vi "Display Item Info.vi"(8 "error in (no error)":errorcluster, 9 "Config":T1, 10 "Control References":T5, 11 "Item in":refnum<class "Item.lvclass">) -> (0 "error out":errorcluster, 3 "Item out":refnum<class "Item.lvclass">)   [LabVIEW 2020, in "VI Properties Editor.lvlib" / "Item.lvclass"]
doc: "Displays the data of <B>Item in</B> to the controls identified by <B>Control References</B>, taking into account <B>Config</B>."
uses:
  Item.lvclass
  CTLs/Main References.ctl
  CTLs/Config.ctl
  CTLs/Filter Info.ctl
  CTLs/Filter Column.ctl
  CTLs/Filter Type.ctl
  VI Properties Editor.lvlib
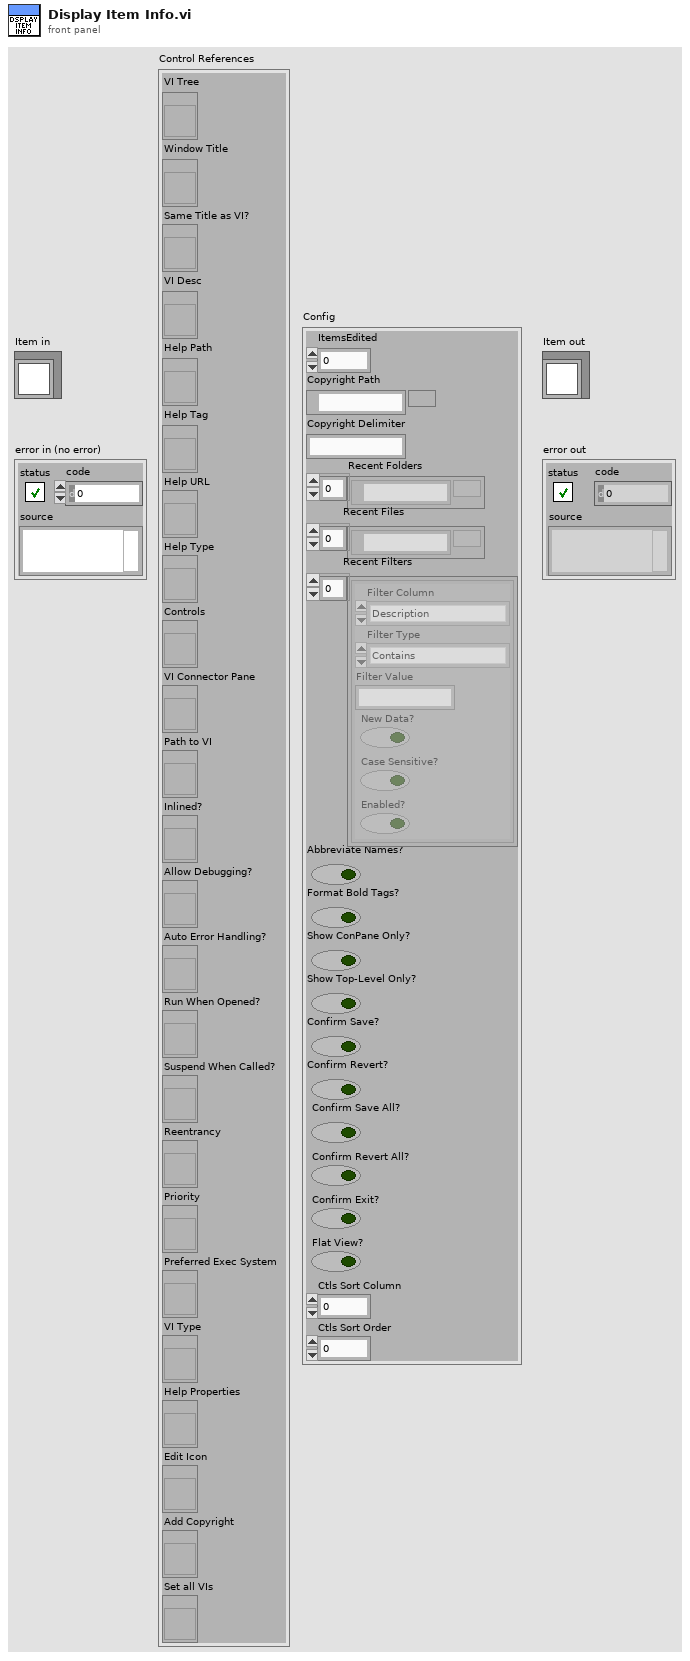
[diagram p1: front panel]
types:
  T1 = typedef "VI Properties Editor.lvlib/Config.ctl" = cluster{"ItemsEdited":u32, "Copyright Path":path, "Copyright Delimiter":string, "Recent Folders":path[], "Recent Files":path[], "Recent Filters":T2[], "Abbreviate Names?":bool, "Format Bold Tags?":bool, "Show ConPane Only?":bool, "Show Top-Level Only?":bool, "Confirm Save?":bool, "Confirm Revert?":bool, "Confirm Save All?":bool, "Confirm Revert All?":bool, "Confirm Exit?":bool, "Flat View?":bool, "Ctls Sort Column":i32, "Ctls Sort Order":i32}
  T2 = typedef "VI Properties Editor.lvlib/Filter Info.ctl" = cluster{"Filter Column":T3, "Filter Type":T4, "Filter Value":string, "New Data?":bool, "Case Sensitive?":bool, "Enabled?":bool}
  T3 = typedef "VI Properties Editor.lvlib/Filter Column.ctl" = enum16{"Name", "Path", "Type", "Window Title", "Description", "Help Path", "Help Tag", "Custom Title?", "Reentrancy", "Inlined?", "Help URL", "Help Type", "Allow Debugging?", "Auto Error Handling?", "Run When Opened?", "Suspend When Called?", "Priority", "Preferred Exec Sytem", "Control Label", "Control Caption", "Control Description", "Control Tip Strip"}
  T4 = typedef "VI Properties Editor.lvlib/Filter Type.ctl" = enum16{"Contains", "Equals", "Starts with", "Ends with", "Is empty", "Does not contain", "Does not equal", "Is not empty"}
  T5 = typedef "VI Properties Editor.lvlib/Main References.ctl" = cluster{"VI Tree":refnum<vi>, "Window Title":refnum<vi>, "Same Title as VI?":refnum<vi>, "VI Desc":refnum<vi>, "Help Path":refnum<vi>, "Help Tag":refnum<vi>, "Help URL":refnum<vi>, "Help Type":refnum<vi>, "Controls":refnum<vi>, "VI Connector Pane":refnum<vi>, "Path to VI":refnum<vi>, "Inlined?":refnum<vi>, "Allow Debugging?":refnum<vi>, "Auto Error Handling?":refnum<vi>, "Run When Opened?":refnum<vi>, "Suspend When Called?":refnum<vi>, "Reentrancy":refnum<vi>, "Priority":refnum<vi>, "Preferred Exec System":refnum<vi>, "VI Type":refnum<vi>, "Help Properties":refnum<vi>, "Edit Icon":refnum<vi>, "Add Copyright":refnum<vi>, "Set all VIs":refnum<vi>}
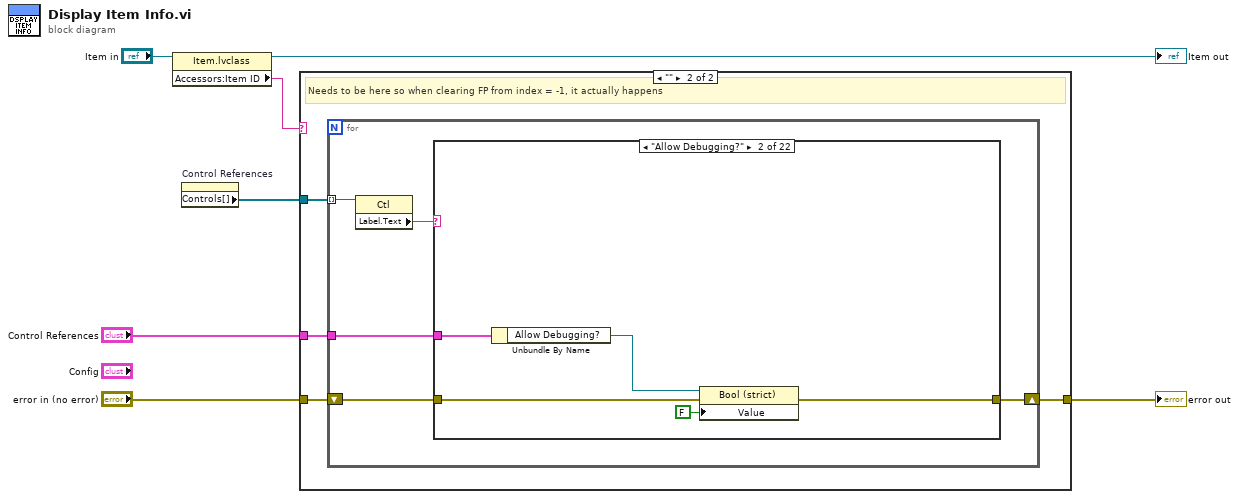
[diagram p0: block diagram]
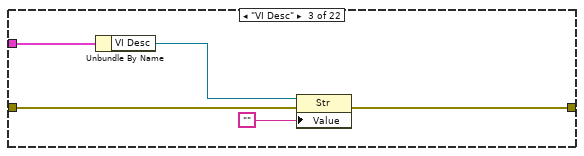
[diagram p4: hidden frame]
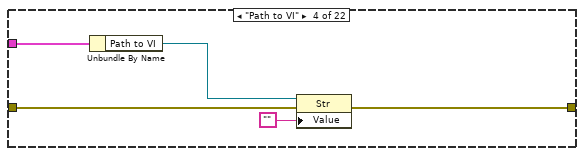
[diagram p5: hidden frame]
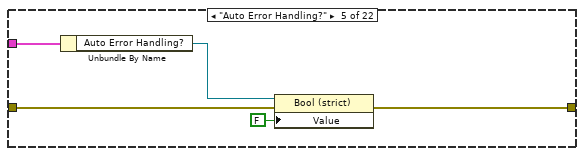
[diagram p6: hidden frame]
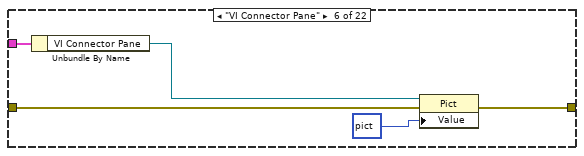
[diagram p7: hidden frame]
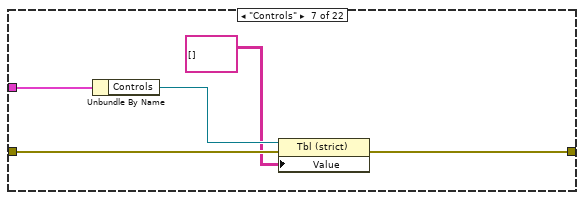
[diagram p8: hidden frame]
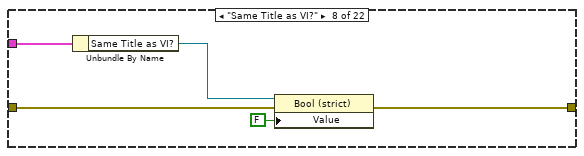
[diagram p9: hidden frame]
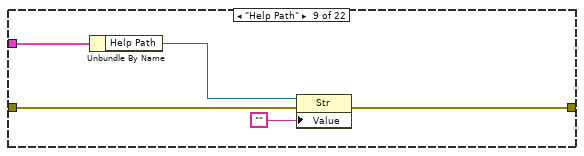
[diagram p10: hidden frame]
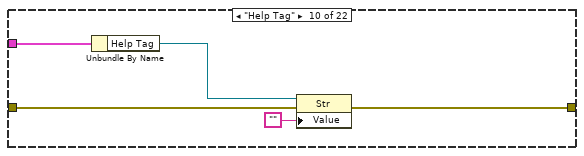
[diagram p11: hidden frame]
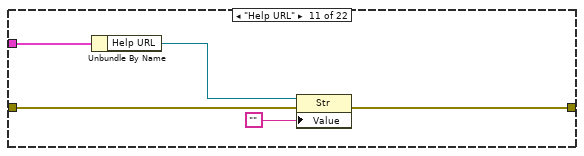
[diagram p12: hidden frame]
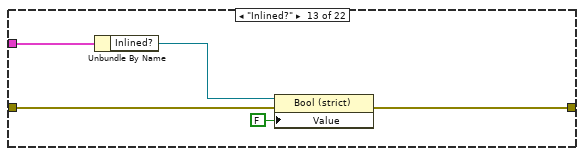
[diagram p14: hidden frame]
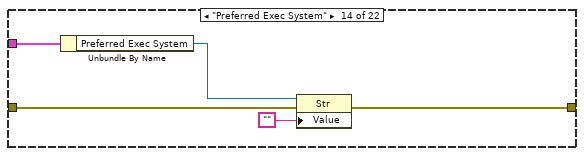
[diagram p15: hidden frame]
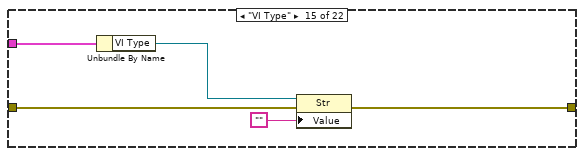
[diagram p16: hidden frame]
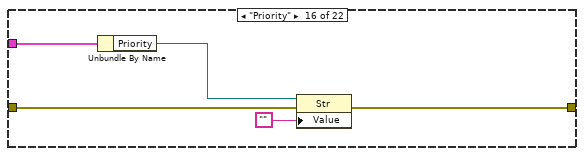
[diagram p17: hidden frame]
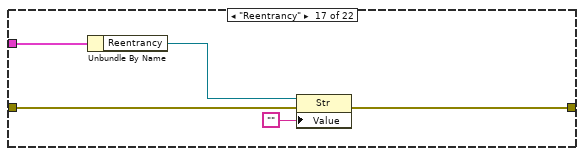
[diagram p18: hidden frame]
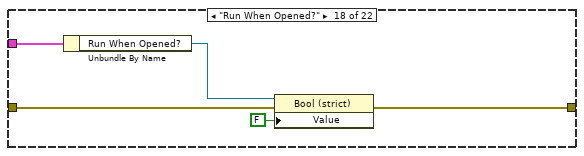
[diagram p19: hidden frame]
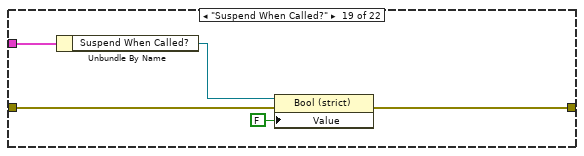
[diagram p20: hidden frame]
diagram:
  n1 = property class="Item.lvclass"(reference="Item in") -> (reference out=→"Item out":refnum<class "Item.lvclass">, "Accessors:Item ID"=w6:string)  [unwired: 1 in, 1 out]
  n2 = property on="Control References" class="Clust (strict)"() -> ("Controls[]"=w2:refnum<vi>[])  [unwired: 2 in, 2 out]
  n3 = case shown="\"\"" w6 {
    tunnel: "Control References" -> [_ w12]
    tunnel: "error in (no error)" -> [w8 w11]
    tunnel: [w8 w10] -> w3
    tunnel: w2 -> [_ w9]
    frame Default {
      # "If Item ID is anything other than empty string, do nothing"
    }
    frame "" {
      # "Needs to be here so when clearing FP from index = -1, it actually happens"
      n4 = for {
        tunnel: w12 -> [w15]
        shift-right: [w16] -> w10
        shift-left: w11 -> [w17]
        tunnel: w9 -> [w14] mode=indexing
        n5 = property class="Ctl"(reference=w14) -> ("Label.Text"=w13:string)  [unwired: 1 in, 2 out]
        n6 = case shown="\"Allow Debugging?\"" w13 {
          tunnel: w17 -> [w18 w21 w26 w31 w36 w41 w46 w51 w56 w61 w66 w69 w72 w77 w82 w87 w92 w97 w102 w105 w108 w111]
          tunnel: w15 -> [_ w23 w28 w33 w38 w43 w48 w53 w58 w63 w68 _ w74 w79 w84 w89 w94 w99 w104 _ w110 _]
          tunnel: [w18 w20 w25 w30 w35 w39 w45 w50 w55 w60 w65 w69 w71 w76 w81 w86 w91 w96 w101 w105 w107 w111] -> w16
          frame Default {
          }
          frame "Allow Debugging?" {
            n7 = Unbundle By Name(w23) -> ("Allow Debugging?"=w22:refnum<vi>)
            n8 = property class="Bool (strict)"(reference=w22, error in=w21, "Value"=FALSE) -> (error out=w20:errorcluster)  [unwired: 1 out]
          }
          frame "VI Desc" {
            n9 = Unbundle By Name(w28) -> ("VI Desc"=w27:refnum<vi>)
            n10 = property class="Str"(reference=w27, error in=w26, "Value"="") -> (error out=w25:errorcluster)  [unwired: 1 out]
          }
          frame "Path to VI" {
            n11 = Unbundle By Name(w33) -> ("Path to VI"=w32:refnum<vi>)
            n12 = property class="Str"(reference=w32, error in=w31, "Value"="") -> (error out=w30:errorcluster)  [unwired: 1 out]
          }
          frame "Auto Error Handling?" {
            n13 = Unbundle By Name(w38) -> ("Auto Error Handling?"=w37:refnum<vi>)
            n14 = property class="Bool (strict)"(reference=w37, error in=w36, "Value"=FALSE) -> (error out=w35:errorcluster)  [unwired: 1 out]
          }
          frame "VI Connector Pane" {
            n15 = Unbundle By Name(w43) -> ("VI Connector Pane"=w42:refnum<vi>)
            n16 = property class="Pict"(reference=w42, error in=w41, "Value"=picture data[5B]) -> (error out=w39:errorcluster)  [unwired: 1 out]
          }
          frame "Controls" {
            n17 = Unbundle By Name(w48) -> ("Controls"=w47:refnum<vi>)
            n18 = property class="Tbl (strict)"(reference=w47, error in=w46, "Value"=string[][] []) -> (error out=w45:errorcluster)  [unwired: 1 out]
          }
          frame "Same Title as VI?" {
            n19 = Unbundle By Name(w53) -> ("Same Title as VI?"=w52:refnum<vi>)
            n20 = property class="Bool (strict)"(reference=w52, error in=w51, "Value"=FALSE) -> (error out=w50:errorcluster)  [unwired: 1 out]
          }
          frame "Help Path" {
            n21 = Unbundle By Name(w58) -> ("Help Path"=w57:refnum<vi>)
            n22 = property class="Str"(reference=w57, error in=w56, "Value"="") -> (error out=w55:errorcluster)  [unwired: 1 out]
          }
          frame "Help Tag" {
            n23 = Unbundle By Name(w63) -> ("Help Tag"=w62:refnum<vi>)
            n24 = property class="Str"(reference=w62, error in=w61, "Value"="") -> (error out=w60:errorcluster)  [unwired: 1 out]
          }
          frame "Help URL" {
            n25 = Unbundle By Name(w68) -> ("Help URL"=w67:refnum<vi>)
            n26 = property class="Str"(reference=w67, error in=w66, "Value"="") -> (error out=w65:errorcluster)  [unwired: 1 out]
          }
          frame "Help Type" {
            # "no point resetting this"
          }
          frame "Inlined?" {
            n27 = Unbundle By Name(w74) -> ("Inlined?"=w73:refnum<vi>)
            n28 = property class="Bool (strict)"(reference=w73, error in=w72, "Value"=FALSE) -> (error out=w71:errorcluster)  [unwired: 1 out]
          }
          frame "Preferred Exec System" {
            n29 = Unbundle By Name(w79) -> ("Preferred Exec System"=w78:refnum<vi>)
            n30 = property class="Str"(reference=w78, error in=w77, "Value"="") -> (error out=w76:errorcluster)  [unwired: 1 out]
          }
          frame "VI Type" {
            n31 = Unbundle By Name(w84) -> ("VI Type"=w83:refnum<vi>)
            n32 = property class="Str"(reference=w83, error in=w82, "Value"="") -> (error out=w81:errorcluster)  [unwired: 1 out]
          }
          frame "Priority" {
            n33 = Unbundle By Name(w89) -> ("Priority"=w88:refnum<vi>)
            n34 = property class="Str"(reference=w88, error in=w87, "Value"="") -> (error out=w86:errorcluster)  [unwired: 1 out]
          }
          frame "Reentrancy" {
            n35 = Unbundle By Name(w94) -> ("Reentrancy"=w93:refnum<vi>)
            n36 = property class="Str"(reference=w93, error in=w92, "Value"="") -> (error out=w91:errorcluster)  [unwired: 1 out]
          }
          frame "Run When Opened?" {
            n37 = Unbundle By Name(w99) -> ("Run When Opened?"=w98:refnum<vi>)
            n38 = property class="Bool (strict)"(reference=w98, error in=w97, "Value"=FALSE) -> (error out=w96:errorcluster)  [unwired: 1 out]
          }
          frame "Suspend When Called?" {
            n39 = Unbundle By Name(w104) -> ("Suspend When Called?"=w103:refnum<vi>)
            n40 = property class="Bool (strict)"(reference=w103, error in=w102, "Value"=FALSE) -> (error out=w101:errorcluster)  [unwired: 1 out]
          }
          frame "Help Properties" {
            # "no point resetting this"
          }
          frame "Window Title" {
            n41 = Unbundle By Name(w110) -> ("Window Title"=w109:refnum<vi>)
            n42 = property class="Str"(reference=w109, error in=w108, "Value"="") -> (error out=w107:errorcluster)  [unwired: 1 out]
          }
          frame "VI Tree" {
            # "Nothing currently done to set the value of the VI Tree programmatically"
          }
        }
      }
    }
  }
  "error out" <- w3
